vi "纳清浊度_所有参数读取.vi"(8 "error in (no error)":errorcluster caption="错误输入（无错误）", 11 "MB session in":refnum<class "MB_Master.lvclass">) -> (0 "error out":errorcluster caption="错误输出", 2 "输出值":T1 {"波特率" items=["4800", "9600", "19200", "38400", "57600", "115200"]}, 3 "MB session out":refnum<class "MB_Master.lvclass">)   [LabVIEW 2016, in "斯坦道多参数.lvlib"]
uses:
  <vilib>/Plasmionique/MB Master/MB_Master/MB_Master.lvclass
  <vilib>/Plasmionique/MB Master/MB Master.lvlib
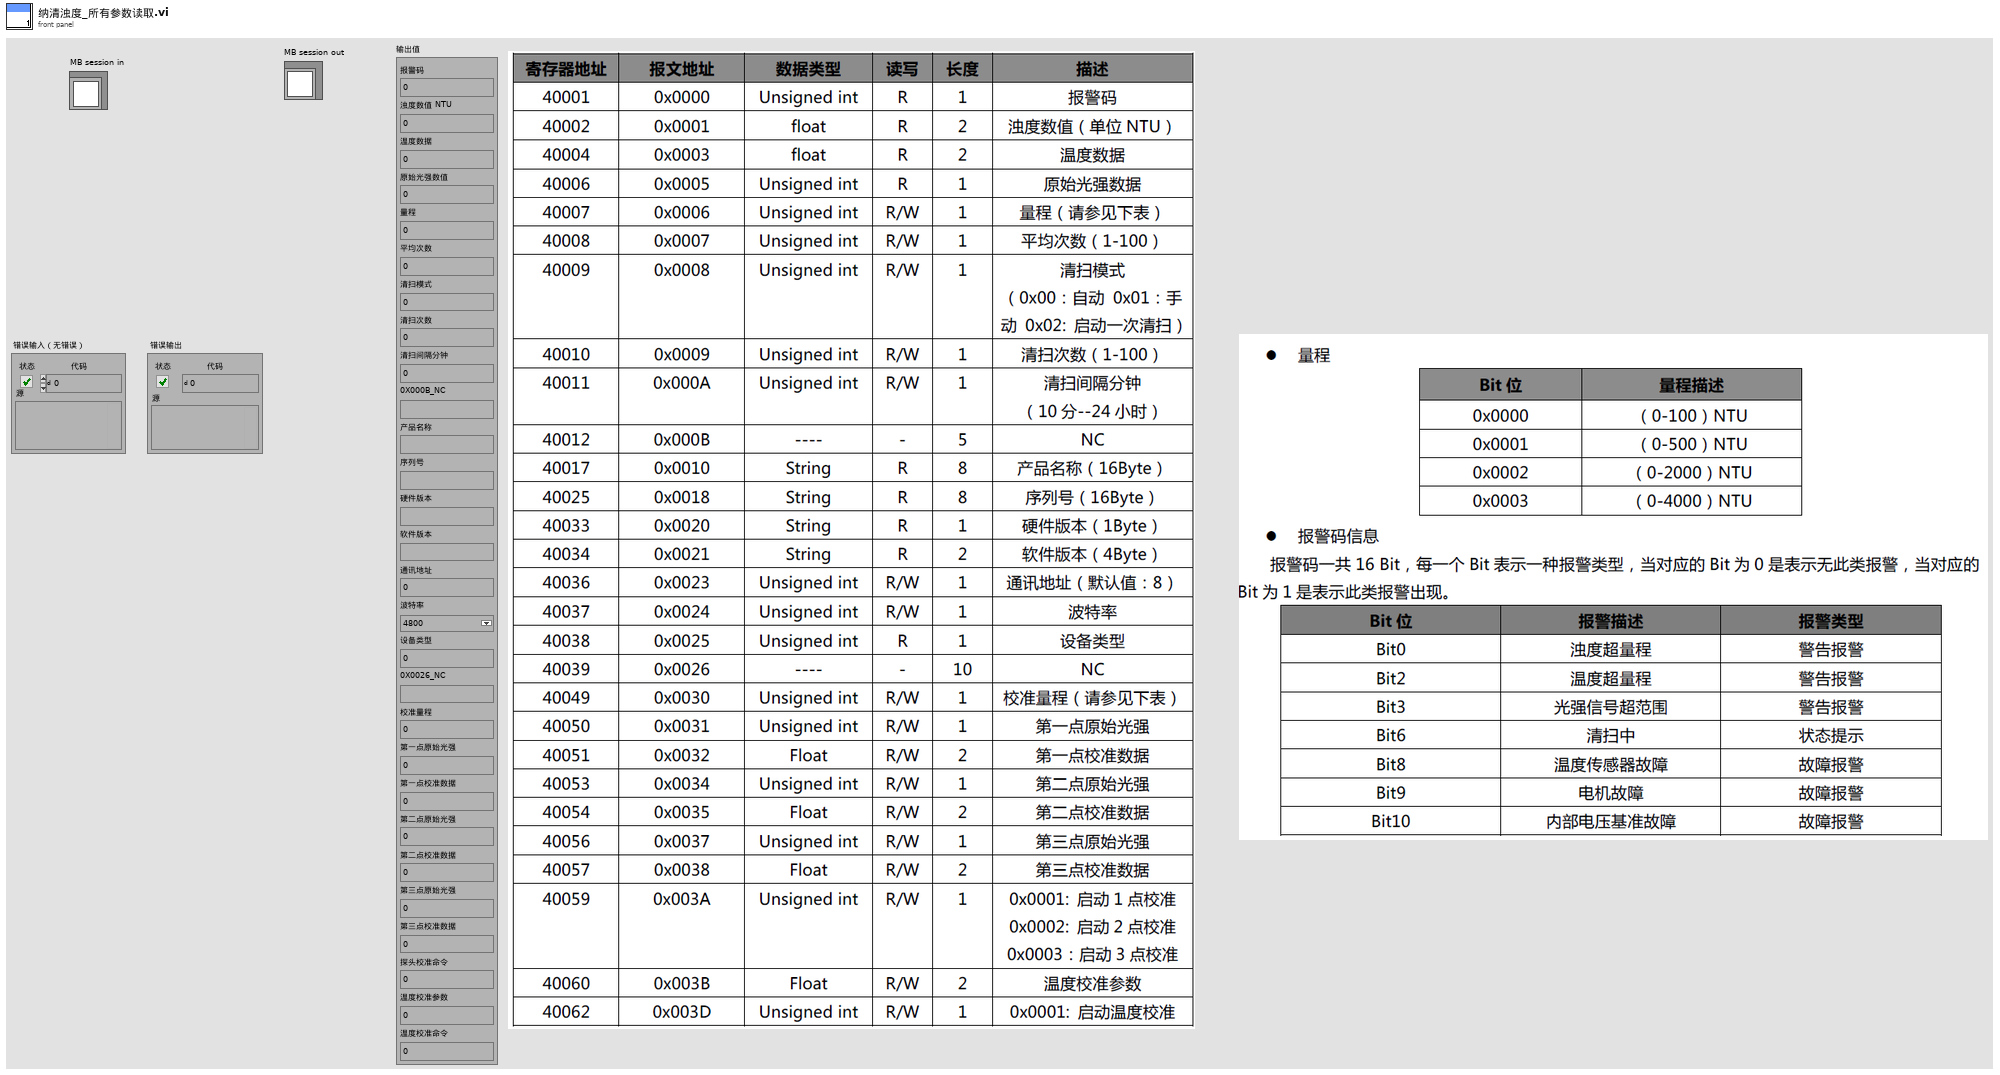
[diagram p1: front panel]
types:
  T1 = cluster{"报警码":u16, "浊度数值 NTU":sgl, "温度数据":sgl, "原始光强数值":u16, "量程":u16, "平均次数":u16, "清扫模式":u16, "清扫次数":u16, "清扫间隔分钟":u16, "0X000B_NC":string, "产品名称":string, "序列号":string, "硬件版本":string, "软件版本":string, "通讯地址":u16, "波特率":u16, "设备类型":u16, "0X0026_NC":string, "校准量程":u16, "第一点原始光强":u16, "第一点校准数据":sgl, "第二点原始光强":u16, "第二点校准数据":sgl, "第三点原始光强":u16, "第三点校准数据":sgl, "探头校准命令":u16, "温度校准参数":sgl, "温度校准命令":u16}
  T2 = cluster{"pH":u32, "DO":u32, "Cond":u32, "Turb":u32, "叶绿素a":u32, "藻密度":u32, "ORP":u32}
  T3 = cluster{u16, "mode":dbl, "数值":sgl, u16, u16, u16, u16, u16, u16, "类型":string, "类型":string, "类型":string, "类型":string, "类型":string, u16, u16, u16, "类型":string, u16, u16, "数值":sgl, u16, "数值":sgl, u16, "数值":sgl, u16, "数值":sgl, u16}
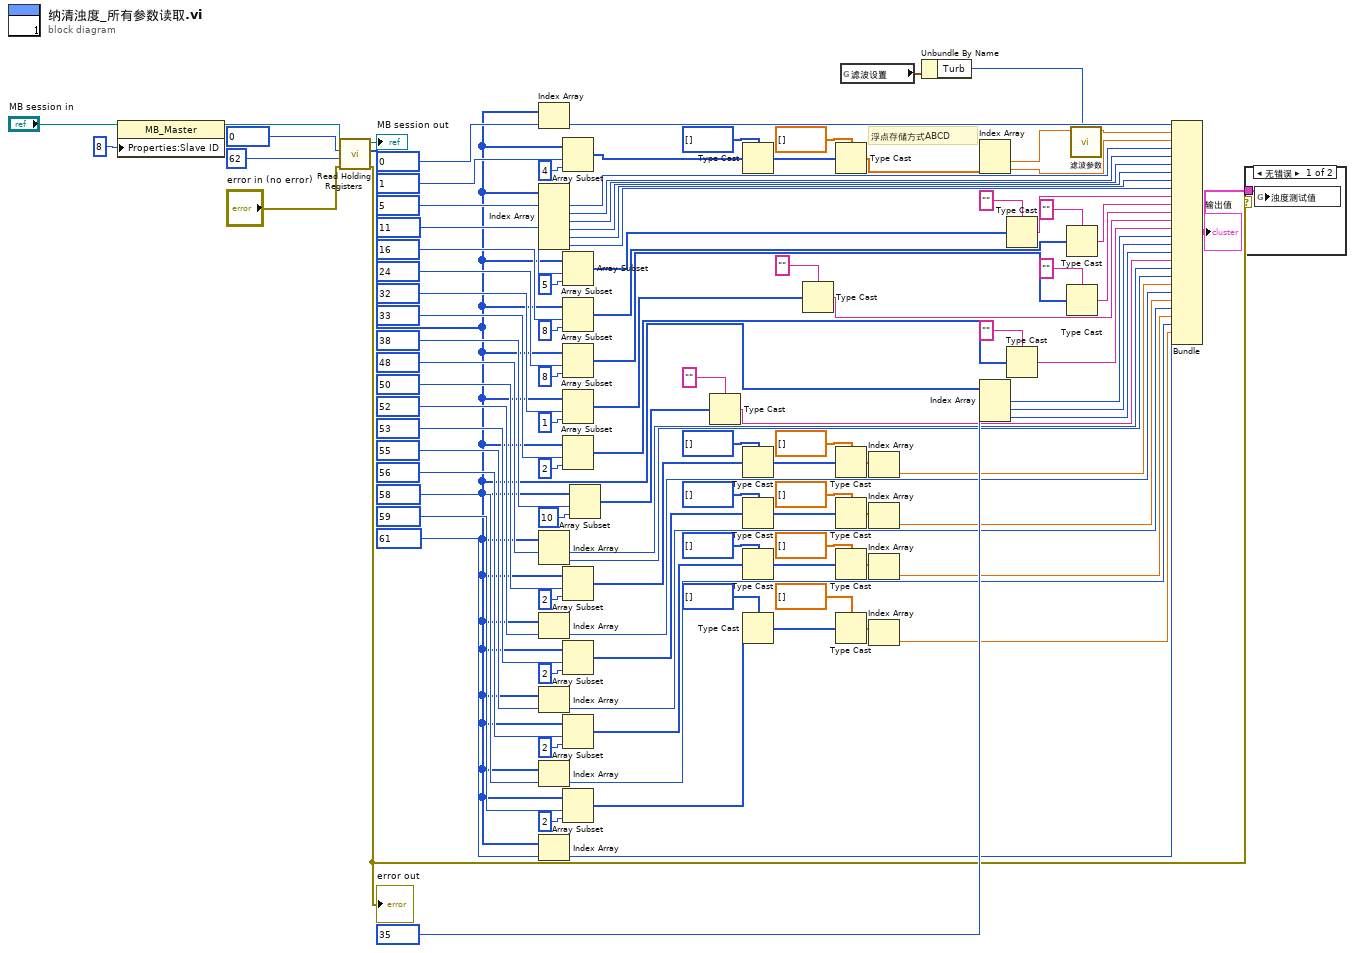
[diagram p0: block diagram]
diagram:
  # "浮点存储方式ABCD"
  n1 = property class="MB_Master"(reference="MB session in", "Properties:Slave ID"=u8 8 ("Slave ID")) -> (reference out=w98:refnum<class "MB_Master.lvclass">)  [unwired: 1 in, 1 out]
  n2 = call <vilib>:"Read Holding Registers.vi"("error in (no error)"="error in (no error)", "quantity"=u16 62, "starting address"=u16 0, "MB session in"=w98) -> ("error out"=w9:errorcluster, "Registers"=w11:u16[], "MB session out"=→"MB session out":refnum<class "MB_Master.lvclass">)  [unwired: 5 in]
  "error out" <- w9
  n3 = Index Array(array=w11, index=u16 0 ("starting address")) -> (element=w106:u16)
  n4 = Index Array(array=w11, index #1=u16 5 ("starting address")) -> (element #1=w93:u16, element #2=w92:u16, element #3=w91:u16, element #4=w90:u16, element #5=w89:u16, element #6=w88:u16)  [unwired: 5 in]
  n5 = Index Array(array=w11, index #1=u16 48 ("starting address")) -> (element #1=w52:u16, element #2=w51:u16)  [unwired: 1 in]
  n6 = Index Array(array=w11, index=u16 52 ("starting address")) -> (element=w34:u16)
  n7 = Index Array(array=w11, index=u16 55 ("starting address")) -> (element=w24:u16)
  n8 = Index Array(array=w11, index=u16 58 ("starting address")) -> (element=w14:u16)
  n9 = Index Array(array=w11, index=u16 61 ("starting address")) -> (element=w10:u16)
  n10 = Array Subset(array=w11, index=u16 1 ("starting address"), length=4 ("长度")) -> (w102:u16[])
  n11 = Array Subset(array=w11, index=u16 11 ("starting address"), length=5 ("长度")) -> (w85:u16[])
  n12 = Array Subset(array=w11, index=u16 16 ("starting address"), length=8 ("长度")) -> (w81:u16[])
  n13 = Array Subset(array=w11, index=u16 24 ("starting address"), length=8 ("长度")) -> (w75:u16[])
  n14 = Array Subset(array=w11, index=u16 32 ("starting address"), length=1 ("长度")) -> (w71:u16[])
  n15 = Array Subset(array=w11, index=u16 33 ("starting address"), length=2 ("长度")) -> (w65:u16[])
  n16 = Array Subset(array=w11, index=u16 50 ("starting address"), length=2 ("长度")) -> (w49:u16[])
  n17 = Array Subset(array=w11, index=u16 53 ("starting address"), length=2 ("长度")) -> (w37:u16[])
  n18 = Array Subset(array=w11, index=u16 56 ("starting address"), length=2 ("长度")) -> (w30:u16[])
  n19 = Array Subset(array=w11, index=u16 59 ("starting address"), length=2 ("长度")) -> (w17:u16[])
  n20 = Array Subset(array=w11, index=u16 38 ("starting address"), length=10 ("长度")) -> (w55:u16[])
  n21 = Type Cast(type="" ("类型"), x=w55) -> (*(type *) &x=w54:string)
  n22 = Type Cast(type=u32[] [] ("数组 2"), x=w102) -> (*(type *) &x=w7:u32[])
  n23 = Type Cast(type=u32[] [] ("数组 2"), x=w49) -> (*(type *) &x=w47:u32[])
  n24 = Type Cast(type=u32[] [] ("数组 2"), x=w37) -> (*(type *) &x=w39:u32[])
  n25 = Type Cast(type=u32[] [] ("数组 2"), x=w30) -> (*(type *) &x=w28:u32[])
  n26 = Type Cast(type=u32[] [] ("数组 2"), x=w17) -> (*(type *) &x=w19:u32[])
  n27 = Type Cast(type="" ("类型"), x=w71) -> (*(type *) &x=w68:string)
  n28 = Type Cast(type=sgl[] [] ("数组 2"), x=w7) -> (*(type *) &x=w101:sgl[])
  n29 = Type Cast(type=sgl[] [] ("数组 2"), x=w47) -> (*(type *) &x=w44:sgl[])
  n30 = Type Cast(type=sgl[] [] ("数组 2"), x=w39) -> (*(type *) &x=w42:sgl[])
  n31 = Type Cast(type=sgl[] [] ("数组 2"), x=w28) -> (*(type *) &x=w25:sgl[])
  n32 = Type Cast(type=sgl[] [] ("数组 2"), x=w19) -> (*(type *) &x=w22:sgl[])
  n33 = global read "断电保存变量.vi" "滤波设置"() -> (w2:T2)
  n34 = Index Array(array=w44) -> (element=w43:sgl)  [unwired: 1 in]
  n35 = Index Array(array=w42) -> (element=w33:sgl)  [unwired: 1 in]
  n36 = Index Array(array=w25) -> (element=w23:sgl)  [unwired: 1 in]
  n37 = Index Array(array=w22) -> (element=w13:sgl)  [unwired: 1 in]
  n38 = Unbundle By Name(w2) -> ("Turb"=w1:u32)
  n39 = Index Array(array=w101) -> (element #1=w4:sgl, element #2=w96:sgl)  [unwired: 2 in]
  n40 = Index Array(array=w11, index #1=u16 35 ("starting address")) -> (element #1=w61:u16, element #2=w60:u16, element #3=w59:u16)  [unwired: 2 in]
  n41 = Type Cast(type="" ("类型"), x=w85) -> (*(type *) &x=w83:string)
  n42 = Type Cast(type="" ("类型"), x=w65) -> (*(type *) &x=w63:string)
  n43 = Type Cast(type="" ("类型"), x=w81) -> (*(type *) &x=w78:string)
  n44 = Type Cast(type="" ("类型"), x=w75) -> (*(type *) &x=w73:string)
  n45 = call "滤波参数.vi"("滤波次数"=w1, "x"=w4) -> ("mode"=w3:dbl)  [unwired: 9 in]
  n46 = Bundle(w106, "mode"=w3, "数值"=w96, w93, w92, w91, w90, w89, w88, "类型"=w83, "类型"=w78, "类型"=w73, "类型"=w68, "类型"=w63, w61, w60, w59, "类型"=w54, w52, w51, "数值"=w43, w34, "数值"=w33, w24, "数值"=w23, w14, "数值"=w13, w10) -> (w8:T3)  [unwired: 1 in]
  "输出值" <- w8
  n47 = case shown="无错误" w9 {
    tunnel: w8 -> [w109 _]
    frame No Error {
      n48 = global write "纳清过程全局变量.vi" "浊度测试值"(w109) -> ()
    }
    frame Error {
    }
  }
